vi "SetFurniture.vi"(8 "error in (no error)":errorcluster, 10 "Furniture":refnum<class "Furniture.lvclass">[](array[class]), 11 "RoomC in":refnum<class "RoomC.lvclass">) -> (0 "error out":errorcluster, 3 "RoomC out":refnum<class "RoomC.lvclass">)   [LabVIEW 2019, in "RoomC.lvclass"]
uses:
  RoomC.lvclass
  Room.lvclass
  Furniture.lvclass
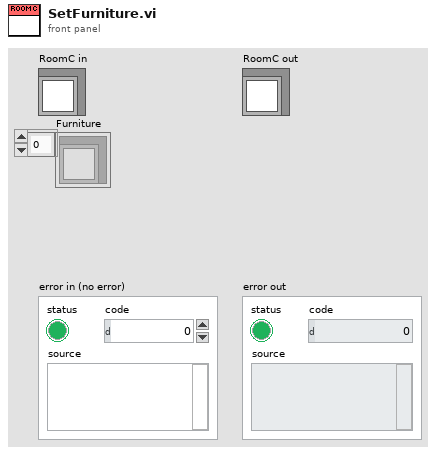
[diagram p1: front panel]
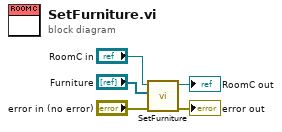
[diagram p0: block diagram]
diagram:
  n1 = call-parent "SetFurniture.vi"("error in (no error)"="error in (no error)", "Furniture"="Furniture", "Room in"="RoomC in") -> ("error out"=→"error out":errorcluster, "Room out"=→"RoomC out":refnum<class "RoomC.lvclass">)  [unwired: 7 in]
